vi "Convert Octave Spectrum to wForm.vi"(0 "Octave Bandwidth":T2(ring), 2 "octave spectra":T1(array[cluster]) {"band power" format="%.2f"; "nominal frequencies [Hz]" format="%.2f"}, 3 "Octave unit labels":string[](array[string]), 4 "Signal Names":string[](array[string]), 5 "Signal Units":string[](array[string])) -> (16 "wForm":waveform(dbl)[](array[waveform]), 18 "Units OUT":string[](array[string]))   [LabVIEW 2022 SP3, in "GSwFormDSP.lvclass"]
uses:
  GSwFormDSP.lvclass
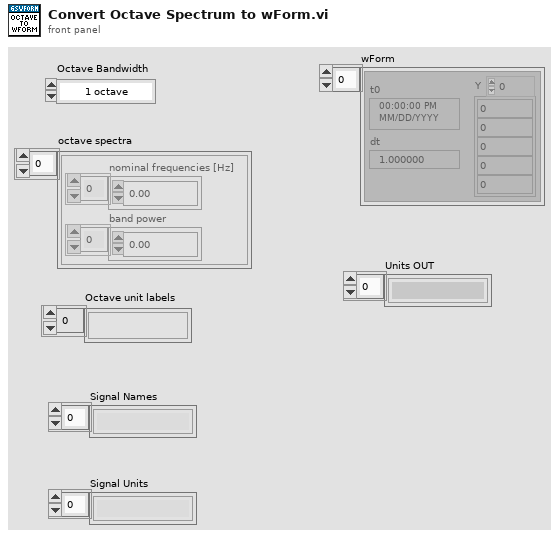
[diagram p1: front panel]
types:
  T1 = cluster{"nominal frequencies [Hz]":dbl[], "band power":dbl[]}[]
  T2 = enum16{"1 octave", "1/3 octave", "1/6 octave", "1/12 octave", "1/24 octave"}
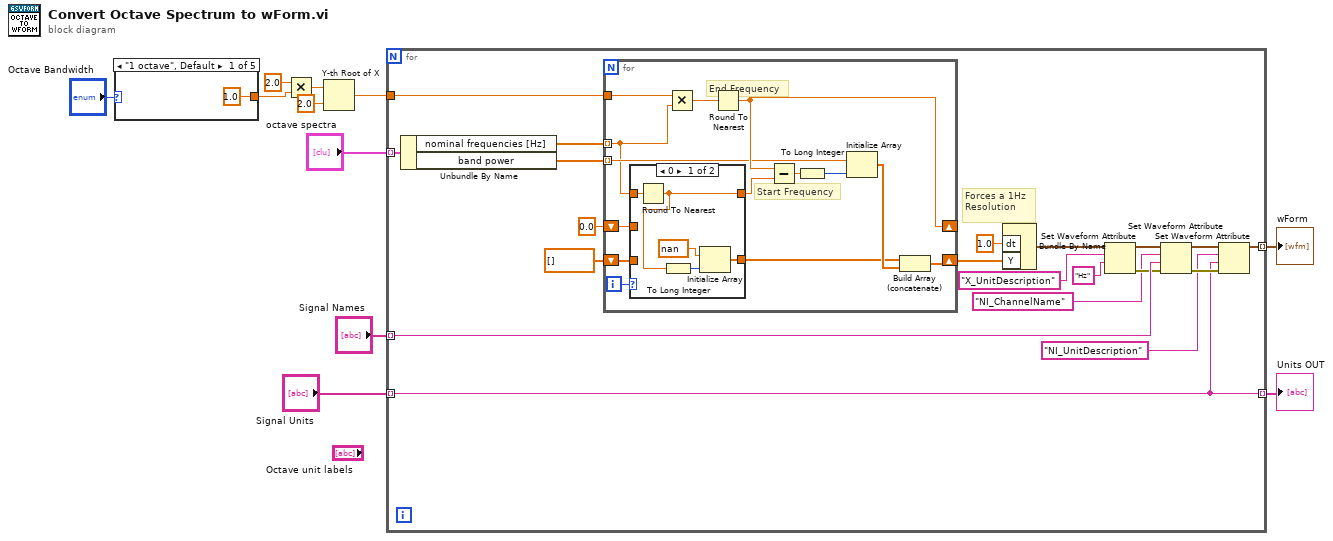
[diagram p0: block diagram]
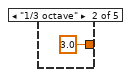
[diagram p2: hidden frame]
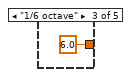
[diagram p3: hidden frame]
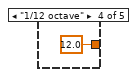
[diagram p4: hidden frame]
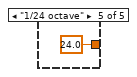
[diagram p5: hidden frame]
diagram:
  n1 = case shown="\"1 octave\", Default" "Octave Bandwidth" {
    tunnel: [1.0 ("x") 3.0 ("x") 6.0 ("x") 12.0 ("x") 24.0 ("x")] -> w11
    frame "1 octave", Default {
    }
    frame "1/3 octave" {
    }
    frame "1/6 octave" {
    }
    frame "1/12 octave" {
    }
    frame "1/24 octave" {
    }
  }
  n2 = Multiply(x=2.0, y=w11) -> (x*y=w6:dbl)
  n3 = Y-th Root of X(1:2.0 ("x"), 2:w6) -> (0:w5:dbl)
  n4 = for {
    tunnel: "octave spectra" -> [w36] mode=indexing
    tunnel: w5 -> [w32]
    tunnel: [w18] -> w4 mode=indexing
    tunnel: "Signal Names" -> [w28] mode=indexing
    tunnel: "Signal Units" -> [w17] mode=indexing
    tunnel: [w17] -> w1 mode=indexing
    # "Forces a 1Hz Resolution"
    n5 = Unbundle By Name(w36) -> ("nominal frequencies [Hz]"=w35:dbl[], "band power"=w34:dbl[])
    n6 = for {
      tunnel: w35 -> [w41] mode=indexing
      tunnel: w34 -> [w45] mode=indexing
      shift-right: [w48] -> _
      shift-left: 0.0 ("x") -> [w39]
      tunnel: w32 -> [w50]
      shift-right: [w44] -> w30
      shift-left: dbl[] [] -> [w37]
      i -> [w42]
      # "Start Frequency"
      # "End Frequency"
      n7 = case shown="0" w42 {
        tunnel: w41 -> [w55 _]
        tunnel: [w53 w57] -> w40
        tunnel: w39 -> [_ w57]
        tunnel: [w51 w56] -> w38
        tunnel: w37 -> [_ w56]
        frame 0 {
          n8 = Round To Nearest(number=w55) -> (nearest integer value=w53:dbl)
          n9 = To Long Integer(number=w53) -> (32bit integer=w54:i32)
          n10 = Initialize Array(nan ("element"), w54) -> (w51:dbl[])
        }
        frame 1, Default {
        }
      }
      n11 = Multiply(x=w50, y=w41) -> (x*y=w49:dbl)
      n12 = Round To Nearest(number=w49) -> (nearest integer value=w48:dbl)
      n13 = Subtract(x=w48, y=w40) -> (x-y=w47:dbl)
      n14 = To Long Integer(number=w47) -> (32bit integer=w46:i32)
      n15 = Initialize Array(w45, w46) -> (w43:dbl[])
      n16 = Build Array (concatenate)(w38, w43) -> (w44:dbl[])
    }
    n17 = Bundle By Name("dt"=1.0, "Y"=w30) -> (w26:waveform(dbl))  [unwired: 1 in]
    n18 = Set Waveform Attribute(5:"Hz", 6:"X_UnitDescription" ("Att - X unit"), 7:w26) -> (0:w27:errorcluster, 3:w25:waveform(dbl))  [unwired: 1 in, 1 out]
    n19 = Set Waveform Attribute(4:w27, 5:w28, 6:"NI_ChannelName" ("Att - wform Name"), 7:w25) -> (0:w21:errorcluster, 3:w20:waveform(dbl))  [unwired: 1 out]
    n20 = Set Waveform Attribute(4:w21, 5:w17, 6:"NI_UnitDescription" ("Att - wform unit"), 7:w20) -> (3:w18:waveform(dbl))  [unwired: 2 out]
  }
  "wForm" <- w4
  "Units OUT" <- w1
